vi "Check PID Gains Cell Edit.vi"(8 "error in (no error)":errorcluster, 10 "Coords":T1, 11 "MulticolumnListbox in":refnum<vi>) -> (0 "error out":errorcluster)   [LabVIEW 2019, in "Control Addon Shared.lvlib"]
uses:
  Control Addon Shared.lvlib
  <vilib>/Utility/miscctls.llb/LVPoint32TypeDef.ctl
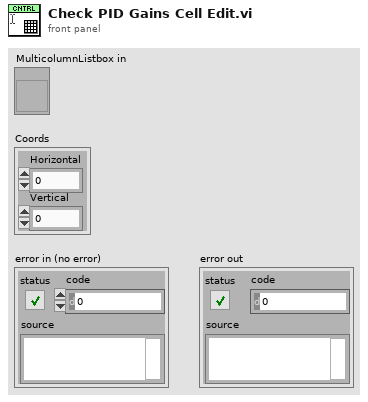
[diagram p1: front panel]
types:
  T1 = typedef "LVPoint32TypeDef.ctl" = cluster{"Horizontal":i32, "Vertical":i32}
  T2 = typedef "LVRowAndColumnTypeDef.ctl" = cluster{"Row":i32, "Column":i32}
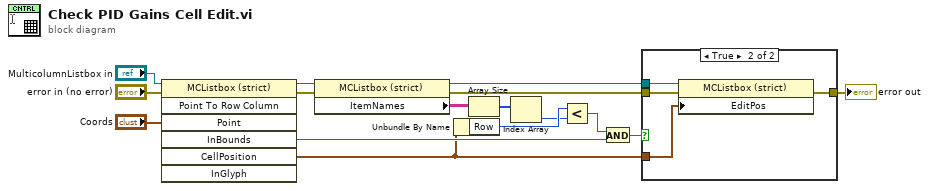
[diagram p0: block diagram]
diagram:
  n1 = invoke class="MCListbox (strict)" method="Point To Row Column"(reference="MulticolumnListbox in", error in="error in (no error)", "Point"="Coords") -> (reference out=w2:refnum<vi>, error out=w12:errorcluster, "InBounds"=w15:bool, "CellPosition"=w14:T2)  [unwired: 4 in, 3 out]
  n2 = property class="MCListbox (strict)"(reference=w2, error in=w12) -> (reference out=w1:refnum<vi>, error out=w13:errorcluster, "ItemNames"=w7:string[][])
  n3 = Unbundle By Name(w14) -> ("Row"=w10:i32)
  n4 = Array Size(array=w7) -> (size(s)=w8:i32[])
  n5 = Index Array(array=w8) -> (element=w9:i32)  [unwired: 1 in]
  n6 = Less?(x=w10, y=w9) -> (x < y?=w11:bool)
  n7 = And(x=w11, y=w15) -> (x .and. y?=w16:bool)
  n8 = case shown="True" w16 {
    tunnel: [w17 w21] -> w6
    tunnel: w1 -> [_ w20]
    tunnel: w13 -> [w17 w19]
    tunnel: w14 -> [_ w18]
    frame False {
    }
    frame True {
      n9 = property class="MCListbox (strict)"(reference=w20, error in=w19, "EditPos"=w18) -> (error out=w21:errorcluster)  [unwired: 1 out]
    }
  }
  "error out" <- w6
